vi "Panel-Sbig.vi"() -> ()   [LabVIEW 2009]
panel:
  in  "Show Cursors":bool=TRUE
  in  "SBIG Name":u16(ring) items=["PI1-SBIG", "PI2-SBIG"]
  in  "Window":bool
  in  "Time":u32
  in  "stop":bool
  out "Graphe intensity":i32[][](graph)
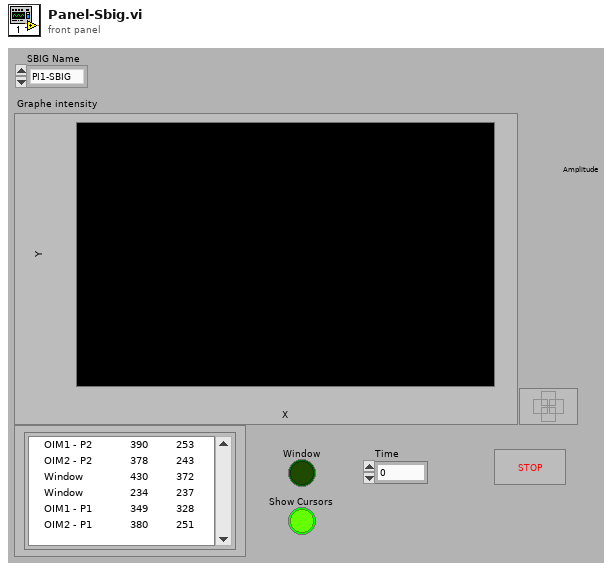
[diagram p1: front panel]
types:
  T1 = cluster{"X0":u16, "Y0":u16, "DX":u16, "DY":u16, "on/off":bool}
  T2 = typedef "LVCursorListTypeDef.ctl" = cluster{"Name":string, "Color":u32, "Style":u8, "Point Style":u8, "Name Visible":bool, "Allow Drag":bool, "Cursor Mode":u32, "Plot":i32, "Index":i32, "Position":cluster{"X":dbl, "Y":dbl}, "X Scale":u32, "Y Scale":u32, "Watch Plots":i32[], "Watch All Plots":bool, "Plot Area":i32, "Label Offset":cluster{"X":dbl, "Y":dbl}}[]
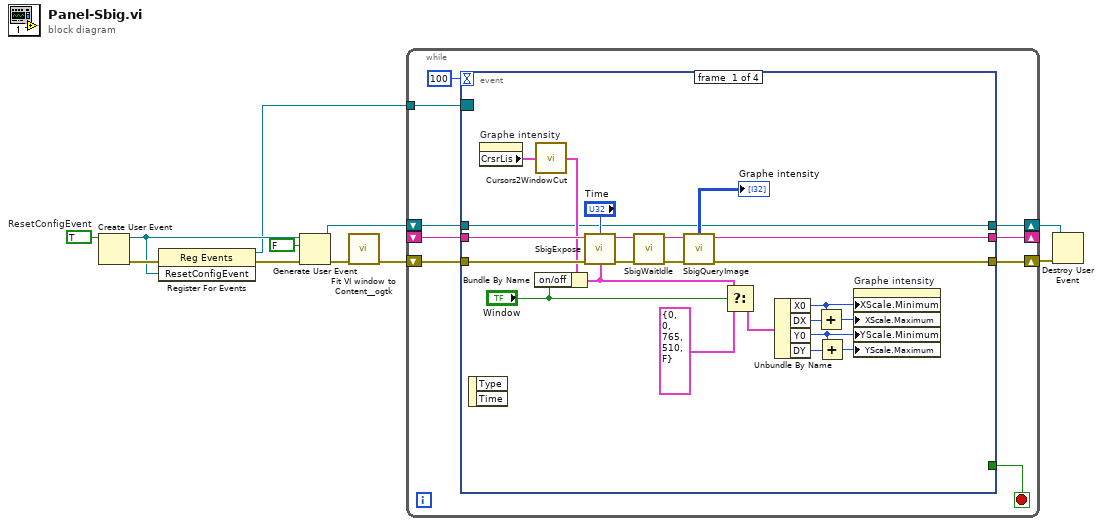
[diagram p0: block diagram]
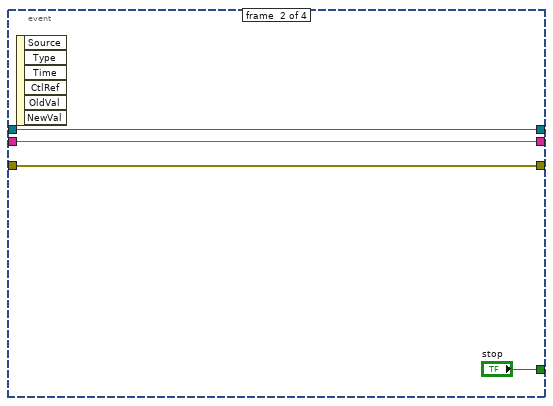
[diagram p2: hidden frame]
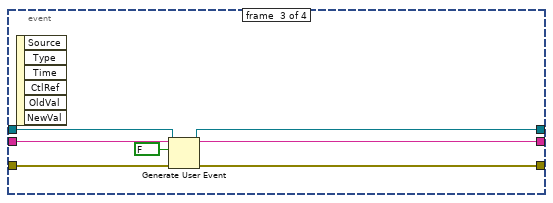
[diagram p3: hidden frame]
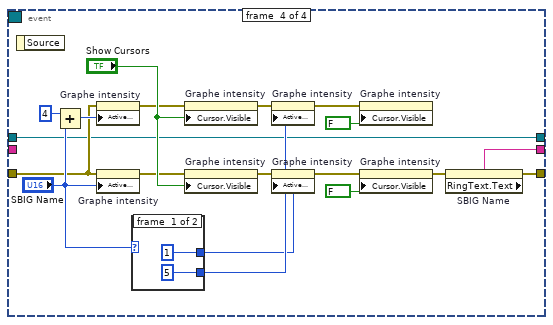
[diagram p4: hidden frame]
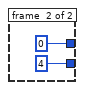
[diagram p5: hidden frame]
diagram:
  w10 = TRUE  # ResetConfigEvent
  n1 = Create User Event(user event datatype=w10) -> (user event=w7:refnum<user-event>, error out=w9:errorcluster)  [unwired: 1 in]
  n2 = register-events(error in=w9, w7) -> (reference out=w5:refnum<event-registration>, error out=w8:errorcluster)  [unwired: 1 in]
  n3 = Generate User Event(user event=w7, event data cluster=FALSE ("event data"), error in=w8) -> (user event out=w3:refnum<user-event>, error out=w4:errorcluster)
  n4 = call <userlib>:"Fit VI window to Content__ogtk.vi"("error in (no error)"=w4) -> ("error out"=w11:errorcluster)  [unwired: 2 in, 4 out]
  n5 = while {
    shift-right: [w18] -> w2
    shift-left: w11 -> [w19]
    shift-right: [w17] -> _
    shift-left: _ -> [w20]
    tunnel: w5 -> [w14]
    shift-right: [w12] -> w1
    shift-left: w3 -> [w13]
    stop <- w15 stop-if-true
    n6 = event shown="[3] <ResetConfigEvent>: User Event" {
      selector: w14 -> [_ _ _ _]
      dyn-events: _ -> [_ _ _ _]
      timeout: 100 -> [_ _ _ _]
      tunnel: w20 -> [w43 w46 w53 _]
      tunnel: w19 -> [w42 w45 w52 w55]
      tunnel: [w41 w45 w51 w57] -> w18
      tunnel: [w39 w46 w53 w56] -> w17
      tunnel: [_ "stop" _ _] -> w15
      tunnel: w13 -> [w21 w44 w49 w54]
      tunnel: [w21 w44 w48 w54] -> w12
      event #0 {
        n7 = event-data() -> ()  [unwired: 3 out]
        n8 = property on="Graphe intensity" class="IntGraph (strict)"() -> ("CrsrLis"=w25:T2)  [unwired: 2 in, 2 out]
        n9 = call "Cursors2WindowCut.vi"("Cursor List"=w25) -> ("Window"=w23:T1)
        n10 = Bundle By Name(cluster=w23, "on/off"="Window") -> (w24:T1)
        n11 = call "SbigExpose.vi"("Time"="Time", "Sbig"=w43, "Window"=w24, "error in (no error)"=w42) -> ("Sbig out"=w37:string, "error out"=w35:errorcluster)  [unwired: 4 out]
        n12 = call "SbigWaitIdle.vi"("error in (no error)"=w35, "Sbig Name"=w37) -> ("error out"=w34:errorcluster, "Sbig Name Out"=w36:string)  [unwired: 8 out]
        n13 = call "SbigQueryImage.vi"("Sbig"=w36, "error in (no error)"=w34) -> ("Sbig out"=w39:string, "Image"=→"Graphe intensity":i32[][], "error out"=w41:errorcluster)  [unwired: 5 out]
        n14 = Select(t=w24, s="Window", f=T1 {"X0"=0, "Y0"=0, "DX"=765, "DY"=510, "on/off"=FALSE} ("Window")) -> (s? t:f=w26:T1)
        n15 = Unbundle By Name(w26) -> ("X0"=w33:u16, "DX"=w32:u16, "Y0"=w29:u16, "DY"=w28:u16)
        n16 = Add(x=w33, y=w32) -> (x+y=w31:u16)
        n17 = Add(x=w29, y=w28) -> (x+y=w30:u16)
        n18 = property on="Graphe intensity" class="IntGraph (strict)"("XScale.Minimum"=w33, "XScale.Maximum"=w31, "YScale.Minimum"=w29, "YScale.Maximum"=w30) -> ()  [unwired: 2 in, 2 out]
      }
      event #1 {
        n19 = event-data() -> ()  [unwired: 7 out]
      }
      event #2 {
        n20 = event-data() -> ()  [unwired: 7 out]
        n21 = Generate User Event(user event=w49, event data cluster=FALSE ("event data"), error in=w52) -> (user event out=w48:refnum<user-event>, error out=w51:errorcluster)
      }
      event #3 {
        n22 = event-data() -> ()  [unwired: 2 out]
        n23 = Add(x=u16 4, y="SBIG Name") -> (x+y=w69:u16)
        n24 = property on="Graphe intensity" class="IntGraph (strict)"(error in=w55, "Active Cursor"=w69) -> (error out=w67:errorcluster)  [unwired: 1 in, 1 out]
        n25 = property on="Graphe intensity" class="IntGraph (strict)"(error in=w55, "Active Cursor"="SBIG Name") -> (error out=w58:errorcluster)  [unwired: 1 in, 1 out]
        n26 = case shown="0, Default" "SBIG Name" {
          tunnel: [1 0] -> w62
          tunnel: [5 4] -> w68
          frame #0 {
          }
          frame #1 {
          }
        }
        n27 = property on="Graphe intensity" class="IntGraph (strict)"(error in=w67, "Cursor.Visible"="Show Cursors") -> (error out=w64:errorcluster)  [unwired: 1 in, 1 out]
        n28 = property on="Graphe intensity" class="IntGraph (strict)"(error in=w58, "Cursor.Visible"="Show Cursors") -> (error out=w61:errorcluster)  [unwired: 1 in, 1 out]
        n29 = property on="Graphe intensity" class="IntGraph (strict)"(error in=w64, "Active Cursor"=w68) -> (error out=w65:errorcluster)  [unwired: 1 in, 1 out]
        n30 = property on="Graphe intensity" class="IntGraph (strict)"(error in=w61, "Active Cursor"=w62) -> (error out=w60:errorcluster)  [unwired: 1 in, 1 out]
        n31 = property on="Graphe intensity" class="IntGraph (strict)"(error in=w65, "Cursor.Visible"=FALSE) -> ()  [unwired: 1 in, 2 out]
        n32 = property on="Graphe intensity" class="IntGraph (strict)"(error in=w60, "Cursor.Visible"=FALSE) -> (error out=w63:errorcluster)  [unwired: 1 in, 1 out]
        n33 = property on="SBIG Name" class="Ring (strict)"(error in=w63) -> (error out=w57:errorcluster, "RingText.Text"=w56:string)  [unwired: 1 in, 1 out]
      }
    }
  }
  n34 = Destroy User Event(user event=w1, error in=w2) -> ()  [unwired: 1 out]
